vi "Poll.Initialize.vi"(7 "FirstCall?":bool, 8 "error in (no error)":errorcluster, 10 "Parameters in":T3 {"Settings"."Data Refs"."Write Refs" format="%.0x"; "Settings"."Data Refs"."Read Refs" format="%.0x"; "Settings"."Write Locations"."DataType" items=["Boolean"=1, "SByte"=2, "Byte"=3, "Int16"=4, "UInt16"=5, "Int32"=6, "UInt32"=7, "Int64"=8, "UInt64"=9, "Float"=10, "Double"=11, "String"=12, "DateTime"=13, "ByteString"=15, "Array of Boolean"=101, "Array of SByte"=102, "Array of Byte"=103, "Array of Int16"=104, "Array of UInt16"=105, "Array of Int32"=106, "Array of UInt32"=107, "Array of Int64"=108, "Array of UInt64"=109, "Array of Float"=110, "Array of Double"=111, "Array of String"=112, "Array of DateTime"=113, "Array of ByteString"=115]}, 11 "Process":refnum<class "Process.lvclass">) -> (0 "error out":errorcluster, 1 "notification":bool, 2 "Parameters out":T3 {"Settings"."Data Refs"."Write Refs" format="%.0x"; "Settings"."Data Refs"."Read Refs" format="%.0x"; "Settings"."Write Locations"."DataType" items=["Boolean"=1, "SByte"=2, "Byte"=3, "Int16"=4, "UInt16"=5, "Int32"=6, "UInt32"=7, "Int64"=8, "UInt64"=9, "Float"=10, "Double"=11, "String"=12, "DateTime"=13, "ByteString"=15, "Array of Boolean"=101, "Array of SByte"=102, "Array of Byte"=103, "Array of Int16"=104, "Array of UInt16"=105, "Array of Int32"=106, "Array of UInt32"=107, "Array of Int64"=108, "Array of UInt64"=109, "Array of Float"=110, "Array of Double"=111, "Array of String"=112, "Array of DateTime"=113, "Array of ByteString"=115]}, 3 "Settings":T1)   [LabVIEW 2019, in "OPC UA Client Addon Engine.lvlib"]
uses:
  OPC UA Client Addon Engine.lvlib
  <vilib>/OPCUA/NI OPC UA Client.lvlib
  Addon Shared/OPC UA Client Addon Shared.lvlib
  <vilib>/NI/NIVS Inline Async API/_VS Inline Async API/Process/Process.lvclass
  <vilib>/NI/NIVS Inline Async API/_Data Access Engine/Data Access Engine/Data Access Engine.lvclass
  Addon Shared/Constants.vi
  <vilib>/NI/NIVS Inline Async API/_Data Access Engine/Data Access Engine/Methods/Write.Lookup.vi
  <vilib>/NI VeriStand/Custom Device API/Data Reference.ctl
  <vilib>/NI VeriStand/Custom Device API/Custom Device API.lvlib
  Addon Shared/Poll.ListProperties.ctl
  Addon Shared/OPCConnection.Properties.ctl
  Addon Shared/Compiled.Settings.ctl
  Types/Poll.Parameters.ctl
  Types/Poll.StateVariables.ctl
  Addon Shared/Tag.WriteProperties.Info.ctl
  Addon Shared/Tags.ReadWriteRefs.ctl
  <vilib>/NI VeriStand/Custom Device API/Custom Device Target Type.ctl
  <vilib>/NI/NIVS Inline Async API/_Data Access Engine/Access Type Classes/Write/Write.lvclass
  <vilib>/NI/NIVS Inline Async API/_Data Access Engine/Data Access Engine/Types/Write.DVR.ctl
  <vilib>/OPCUA/controls/Subscription ID.ctl
  <vilib>/OPCUA/controls/OPC UA StatusCode.ctl
  <vilib>/OPCUA/controls/Data Type.ctl
  <vilib>/OPCUA/controls/NodeId.ctl
  <vilib>/OPCUA/controls/Subscription Data Change.ctl
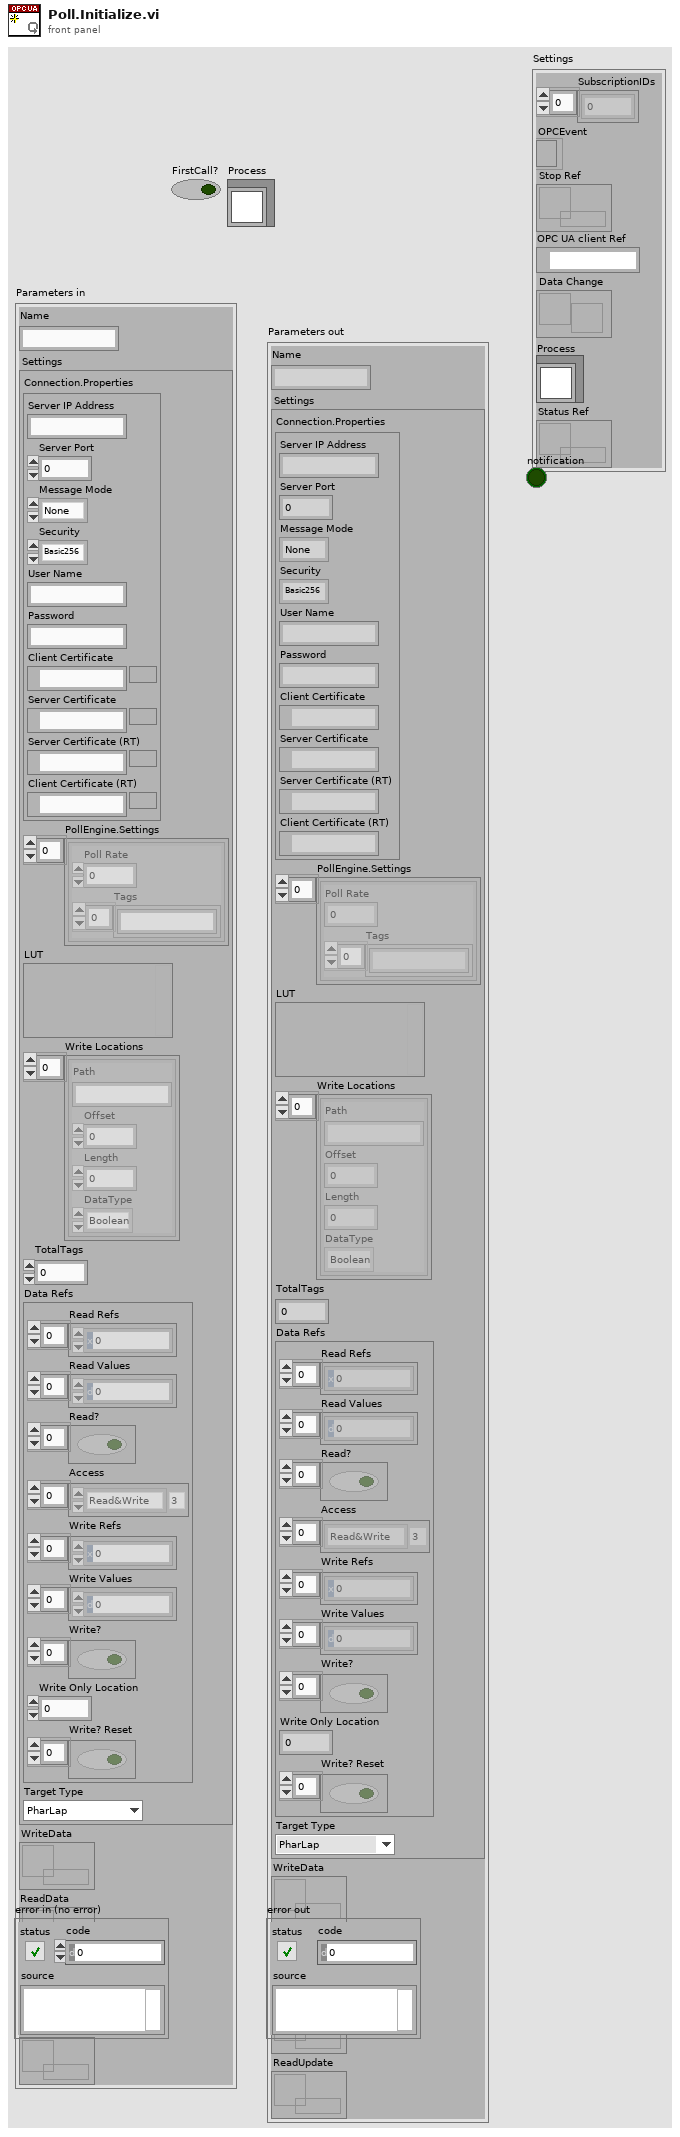
[diagram p1: front panel]
types:
  T1 = typedef "OPC UA Client Addon Engine.lvlib/Poll.StateVariables.ctl" = cluster{"SubscriptionIDs":u32[], "OPCEvent":refnum<event-registration>, "Stop Ref":refnum<data-value>, "OPC UA client Ref":refnum<k21>, "Data Change":refnum<user-event>, "Process":refnum<class "Process.lvclass">, "Status Ref":T2}
  T2 = typedef "Data Access Engine.lvlib/Data Access Engine.lvclass/Write.DVR.ctl" = refnum<data-value>
  T3 = typedef "OPC UA Client Addon Engine.lvlib/Poll.Parameters.ctl" = cluster{"Name":string, "Settings":T4, "WriteData":refnum<k33>, "ReadData":refnum<k33>, "WriteUpdate":refnum<k33>, "ReadUpdate":refnum<k33>}
  T4 = typedef "OPC UA Client Addon Shared.lvlib/Compiled.Settings.ctl" = cluster{"Connection.Properties":T5, "PollEngine.Settings":T6[], "LUT":variant, "Write Locations":T7[], "TotalTags":u32, "Data Refs":T8, "Target Type":T10}
  T5 = typedef "OPC UA Client Addon Shared.lvlib/OPCConnection.Properties.ctl" = cluster{"Server IP Address":string, "Server Port":u16, "Message Mode":enum16{"None", "Sign", "Sign and Encrypt"}, "Security":enum16{"Basic256", "Basic128Rsa15"}, "User Name":string, "Password":string, "Client Certificate":path, "Server Certificate":path, "Server Certificate (RT)":path, "Client Certificate (RT)":path}
  T6 = typedef "OPC UA Client Addon Shared.lvlib/Poll.ListProperties.ctl" = cluster{"Poll Rate":dbl, "Tags":string[]}
  T7 = typedef "OPC UA Client Addon Shared.lvlib/Tag.WriteProperties.Info.ctl" = cluster{"Path":string, "Offset":i32, "Length":i32, "DataType":u32}
  T8 = typedef "OPC UA Client Addon Shared.lvlib/Tags.ReadWriteRefs.ctl" = cluster{"Read Refs":T9[], "Read Values":dbl[], "Read?":bool[], "Access":enum8{"Null", "Read", "Write", "Read&Write"}[], "Write Refs":T9[], "Write Values":dbl[], "Write?":bool[], "Write Only Location":u32, "Write? Reset":bool[]}
  T9 = typedef "Custom Device API.lvlib/Data Reference.ctl" = i32
  T10 = typedef "Custom Device API.lvlib/Custom Device Target Type.ctl" = enum16{"PharLap", "VxWorks", "Windows", "Linux_32_ARM", "Linux_x64"}
  T11 = cluster{"message mode":enum16{"None", "Sign", "Sign and Encrypt"}, "security":enum16{"Basic256", "Basic128Rsa15"}}
  T12 = typedef "OPC UA Client Refnum.ctl" = refnum<k21>
  T13 = typedef "Subscription ID.ctl" = u32
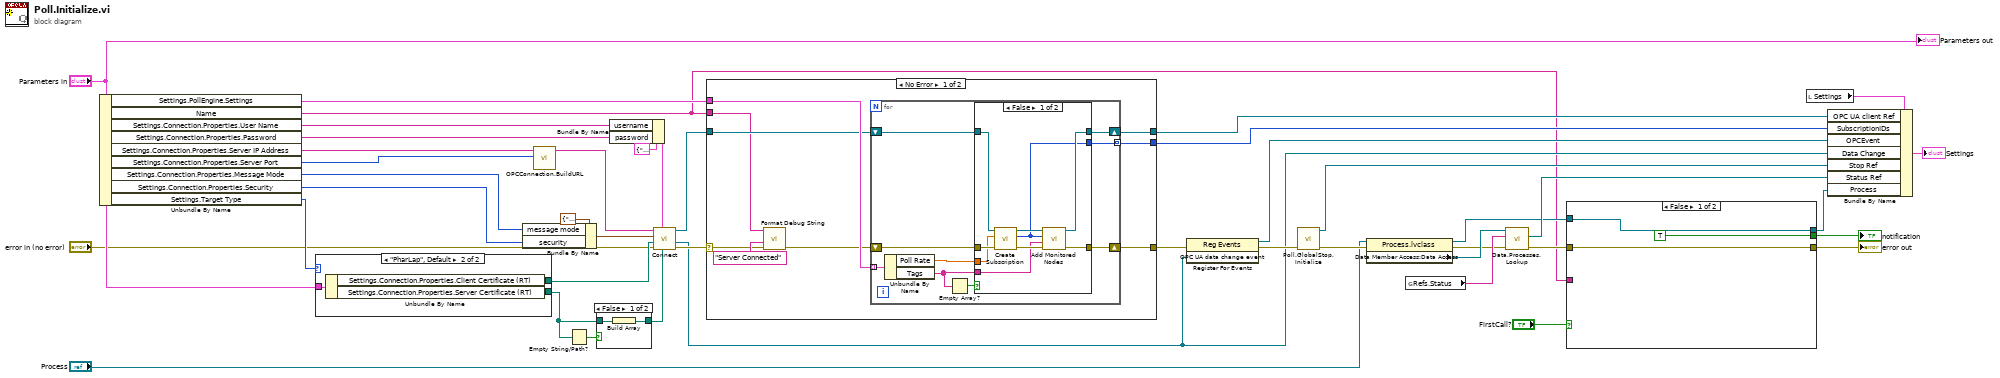
[diagram p0: block diagram]
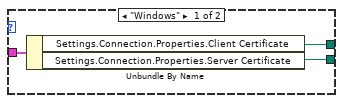
[diagram p5: hidden frame]
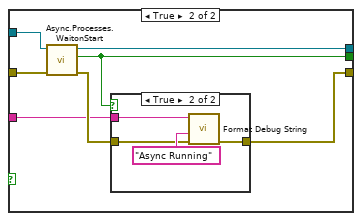
[diagram p6: hidden frame]
diagram:
  n1 = Unbundle By Name("Parameters in") -> ("Settings.PollEngine.Settings"=w24:T6[], "Name"=w1:string, "Settings.Connection.Properties.User Name"=w30:string, "Settings.Connection.Properties.Password"=w29:string, "Settings.Connection.Properties.Server IP Address"=w34:string, "Settings.Connection.Properties.Server Port"=w33:u16, "Settings.Connection.Properties.Message Mode"=w28:enum16{"None", "Sign", "Sign and Encrypt"}, "Settings.Connection.Properties.Security"=w27:enum16{"Basic256", "Basic128Rsa15"}, "Settings.Target Type"=w23:T10)
  n2 = case shown="\"PharLap\", Default" w23 {
    tunnel: [w46 w49] -> w26
    tunnel: [w45 w48] -> w32
    tunnel: "Parameters in" -> [w44 w47]
    frame "Windows" {
      n3 = Unbundle By Name(w44) -> ("Settings.Connection.Properties.Client Certificate"=w46:path, "Settings.Connection.Properties.Server Certificate"=w45:path)
    }
    frame "PharLap", Default {
      n4 = Unbundle By Name(w47) -> ("Settings.Connection.Properties.Client Certificate (RT)"=w49:path, "Settings.Connection.Properties.Server Certificate (RT)"=w48:path)
    }
  }
  n5 = Bundle By Name(cluster=T11 {"message mode"=enum."Sign", "security"=enum."Basic256"} ("security policy"), "message mode"=w28, "security"=w27) -> (w35:T11)
  n6 = call "OPCConnection.BuildURL.vi"("Server Port"=w33, "Server IP Address"=w34) -> ("OPC Path"=w9:string)  [unwired: 9 in]
  n7 = Empty String/Path?(string/path=w32) -> (empty?=w25:bool)
  n8 = case shown="False" w25 {
    tunnel: [w51 _] -> w31
    tunnel: w32 -> [w50 _]
    frame False {
      n9 = Build Array(w50) -> (w51:path[])
    }
    frame True {
    }
  }
  n10 = Bundle By Name(cluster=cluster{"username":string, "password":string} {"username"="", "password"=""} ("username/password"), "username"=w30, "password"=w29) -> (w37:cluster{"username":string, "password":string})
  n11 = call <vilib>:"Connect.vi"("trusted server certificates"=w31, "username/password"=w37, "error in (no error)"="error in (no error)", "client certificate file"=w26, "security policy"=w35, "server endpoint URL"=w9) -> ("error out"=w7:errorcluster, "OPC UA data change event"=w4:refnum<user-event>, "OPC UA client refnum out"=w22:T12)  [unwired: 3 in]
  n12 = case shown="No Error" w7 {
    selector: w7 -> [w54 w82]
    tunnel: [w60 _] -> w41
    tunnel: w24 -> [w59 _]
    tunnel: w22 -> [w58 w81]
    tunnel: [w57 w81] -> w20
    tunnel: [w56 w82] -> w8
    tunnel: w1 -> [w52 _]
    frame No Error {
      n13 = call "Format Debug String.vi"("error in (no error)"=w54, "State"="Server Connected", "Name"=w52) -> ("error out"=w53:errorcluster)  [unwired: 8 in]
      n14 = for {
        tunnel: [w67] -> w60 mode=indexing
        tunnel: w59 -> [w64] mode=indexing
        shift-right: [w68] -> w56
        shift-left: w53 -> [w65]
        shift-right: [w69] -> w57
        shift-left: w58 -> [w66]
        n15 = Unbundle By Name(w64) -> ("Poll Rate"=w63:dbl, "Tags"=w61:string[])
        n16 = Empty Array?(array=w61) -> (empty?=w62:bool)
        n17 = case shown="False" w62 {
          tunnel: [w76 w80] -> w69
          tunnel: [w75 w79] -> w68
          tunnel: [w74 _] -> w67
          tunnel: w66 -> [w73 w80]
          tunnel: w65 -> [w72 w79]
          tunnel: w63 -> [w71 _]
          tunnel: w61 -> [w70 _]
          frame False {
            n18 = call <vilib>:"Create Subscription.vi"("error in (no error)"=w72, "publishing interval (1000 ms)"=w71, "OPC UA client refnum in"=w73) -> ("error out"=w77:errorcluster, "subscription ID out"=w74:T13, "OPC UA client refnum out"=w78:T12)  [unwired: 4 in, 2 out]
            n19 = call <vilib>:"Add Monitored Nodes.vi"("error in (no error)"=w77, "node IDs"=w70, "subscription ID in"=w74, "OPC UA client refnum in"=w78) -> ("error out"=w75:errorcluster, "OPC UA client refnum out"=w76:T12)  [unwired: 5 in, 1 out]
          }
          frame True {
          }
        }
      }
    }
    frame Error {
    }
  }
  n20 = register-events(error in=w8, w4) -> (reference out=w3:refnum<event-registration>, error out=w42:errorcluster)  [unwired: 1 in]
  n21 = call "Poll.GlobalStop.Initialize.vi"("error in (no error)"=w42) -> ("error out"=w14:errorcluster, "Stop Ref"=w40:refnum<data-value>)  [unwired: 9 in]
  n22 = property class="Process.lvclass"(reference="Process", error in=w14) -> (reference out=w10:refnum<class "Process.lvclass">, error out=w13:errorcluster, "Data Member Access:Data Access"=w17:refnum<class "Data Access Engine.lvclass">)
  n23 = global read "Constants.vi" "Refs.Status"() -> (w16:string)
  n24 = call-poly <vilib>:"Data.Processes.Lookup.vi"("error in (no error)"=w13, "Name"=w16, "Data Access API in"=w17) -> ("error out"=w15:errorcluster, "Ref"=w12:T2)  [unwired: 5 in, 2 out]
  n25 = case shown="False" "FirstCall?" {
    tunnel: [w85 w87] -> w43
    tunnel: [TRUE ("notification") w89] -> w39
    tunnel: w15 -> [w85 w91]
    tunnel: w10 -> [w83 w92]
    tunnel: [w83 w90] -> w18
    tunnel: w1 -> [_ w86]
    frame False {
    }
    frame True {
      n26 = call <vilib>:"Async.Processes.WaitonStart.vi"("error in (no error)"=w91, "Process"=w92) -> ("error out"=w88:errorcluster, "Execute"=w89:bool, "Process out"=w90:refnum<class "Process.lvclass">)  [unwired: 7 in]
      n27 = case shown="True" w89 {
        tunnel: w88 -> [w93 w96]
        tunnel: [w93 w95] -> w87
        tunnel: w86 -> [_ w94]
        frame False {
        }
        frame True {
          n28 = call "Format Debug String.vi"("error in (no error)"=w96, "State"="Async Running", "Name"=w94) -> ("error out"=w95:errorcluster)  [unwired: 8 in]
        }
      }
    }
  }
  "error out" <- w43
  "notification" <- w39
  n29 = local read "Settings"() -> (w6:T1)
  n30 = Bundle By Name(cluster=w6, "OPC UA client Ref"=w20, "SubscriptionIDs"=w41, "OPCEvent"=w3, "Data Change"=w4, "Stop Ref"=w40, "Status Ref"=w12, "Process"=w18) -> (→"Settings":T1)
  "Parameters out" <- "Parameters in"
